vi "JH kpfm-z steps upward.vi"() -> ()   [LabVIEW 2014]
uses:
  <userlib>/Nanonis Prog Interface V5/Nanonis Prog Interface.lvlib
panel:
  out "Z starting position  (m)":sgl format="%#_6p"
  in  "Z increment (m)":sgl format="%#_6p"
  in  "steps upward":i32
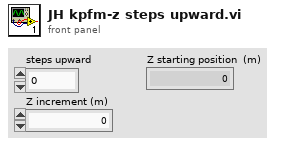
[diagram p1: front panel]
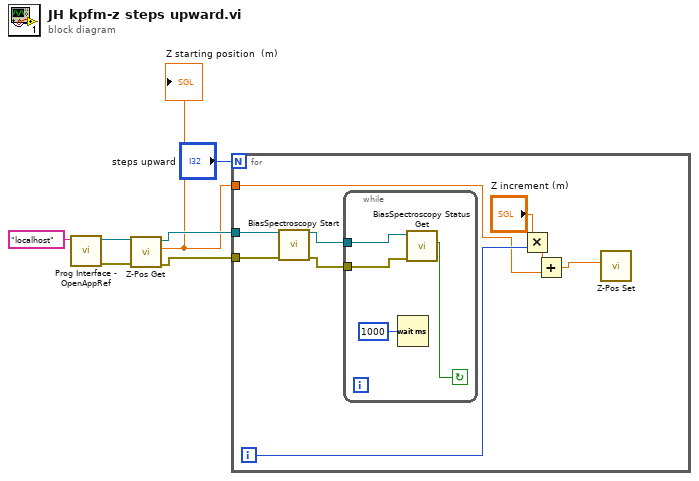
[diagram p0: block diagram]
diagram:
  n1 = call <userlib>:"Prog Interface - OpenAppRef.vi"("Machine name (local machine IP)"="localhost") -> ("Error out"=w5:errorcluster, "Application reference"=w6:refnum<vi>)  [unwired: 5 in]
  n2 = call <userlib>:"Z-Pos Get.vi"("error in (no error)"=w5, "Application ref in"=w6) -> ("error out"=w2:errorcluster, "Z position (m)"=w1:sgl, "Application ref out"=w3:refnum<vi>)  [unwired: 7 in]
  "Z starting position  (m)" <- w1
  n3 = for {
    N: "steps upward" -> [_]
    tunnel: w3 -> [w15]
    tunnel: w2 -> [w14]
    tunnel: w1 -> [w8]
    i -> [w9]
    n4 = call <userlib>:"BiasSpectroscopy Start.vi"("Application ref in"=w15, "Error in (no error)"=w14) -> ("Application ref out"=w13:refnum<vi>, "Error out"=w12:errorcluster)  [unwired: 9 in, 3 out]
    n5 = while {
      tunnel: w13 -> [w20]
      tunnel: w12 -> [w19]
      stop <- w18 continue-if-true
      n6 = Wait (ms)(milliseconds to wait=u32 1000) -> ()  [unwired: 1 out]
      n7 = call <userlib>:"BiasSpectroscopy Status Get.vi"("Error in (no error)"=w19, "Application ref in"=w20) -> ("Running?"=w18:bool)  [unwired: 5 in, 2 out]
    }
    n8 = Multiply(x="Z increment (m)", y=w9) -> (x*y=w10:sgl)
    n9 = Add(x=w10, y=w8) -> (x+y=w11:sgl)
    n10 = call <userlib>:"Z-Pos Set.vi"("Z position (m)"=w11) -> ()  [unwired: 9 in, 2 out]
  }
